vi "FM Ch Time Out En.vi"(9 "Enabled":u8, 10 "Channel":u8, 11 "devId":i32) -> (2 "devId out":i32, 3 "function return":i32)   [LabVIEW 2013, in "CHR34XXX.lvlib"]
doc: "DLL BOOL __stdcall CHR34XXX_FM_Ch_TimeOutEn(IN int devId,IN BYTE Channel,IN BYTE Enabled);"
uses:
  CHR34XXX.lvlib
  CHR34XXX.dll
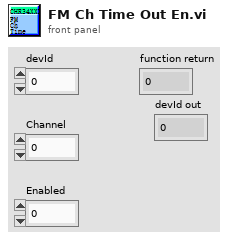
[diagram p1: front panel]
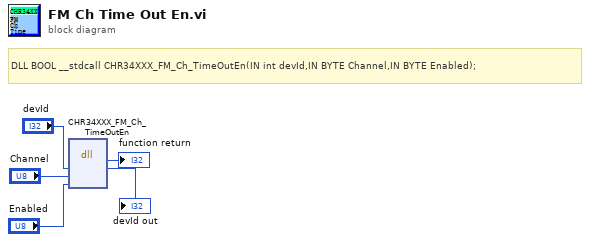
[diagram p0: block diagram]
diagram:
  # "DLL BOOL __stdcall CHR34XXX_FM_Ch_TimeOutEn(IN int devId,IN BYTE Channel,IN BYTE Enabled);"
  n1 = dll-call lib="C:/Users/Administrator/Desktop/CHR34XXX_lv/lv_lib/CHR34XXX.*" fn="CHR34XXX_FM_Ch_TimeOutEn"("devId"="devId", "Channel"="Channel", "Enabled"="Enabled") -> (→"function return":i32, "devId"=→"devId out":i32)  [unwired: 5 in, 2 out]
